vi "Pack for gRPC.vi"(8 "error in":errorcluster, 9 "configuration / results":enum16{"Configuration", "Results"}(ring), 10 "data value":variant, 11 "measurement customizations in":refnum<class "Measurement Plugin.lvclass">) -> (0 "error out":errorcluster, 2 "any":T1, 3 "measurement customizations out":refnum<class "Measurement Plugin.lvclass">)   [LabVIEW 2021, in "Waveform Mode_Channel Ganging.lvlib" / "Measurement Plugin.lvclass"]
uses:
  Measurement Plugin.lvclass
  <vilib>/gRPC/LabVIEW gRPC Library/Shared/Any.ctl
  C:/Program Files/National Instruments/LabVIEW 2021/vi.lib/Plug-In SDKs/Measurements/Measurement Plugin Service/Measurement Plugin Service.lvclass
  Measurement Configuration.ctl
  Measurement Results.ctl
  2eca732d-dbaa-43bf-a7dd-ede2da65bc1b.vi
  a6012965-5700-4384-8228-972e71b6560c.vi
  <vilib>/gRPC/LabVIEW gRPC Library/Server API/Translate Protobuf Error.vi
  <vilib>/AdvancedString/1D String Array to Delimited String.vi
  <vilib>/gRPC/LabVIEW gRPC Library/Server API/Server/Get Server DLL Path.vi
  Measurement Plugin.lvclass/Measurement Plugin.ctl
  Waveform Mode_Channel Ganging.lvlib
  <vilib>/Plug-In SDKs/Measurements/Measurement Plugin Service/Measurement Plugin Service.lvclass
  <vilib>/gRPC/LabVIEW gRPC Library/grpc-lvsupport-release.lvlib
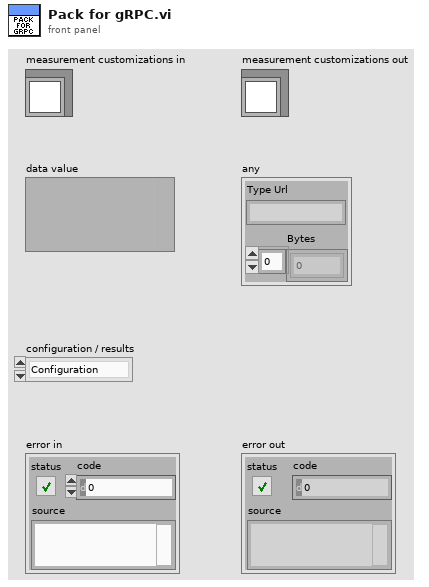
[diagram p1: front panel]
types:
  T1 = typedef "grpc-lvsupport-release.lvlib/Any.ctl" = cluster{"Type Url":string, "Bytes":u8[]}
  T2 = typedef "grpc-lvsupport-release.lvlib/grpcId.ctl" = u64
  T3 = typedef "Waveform Mode_Channel Ganging.lvlib/Measurement Configuration.ctl" = cluster{"Source voltage/current gain bandwidths":dbl[], "Source voltage/current compensation frequencies":dbl[], "Source voltage/current pole-zero ratios":dbl[], "Load voltage/current gain bandwidths":dbl[], "Load voltage/current compensation frequencies":dbl[], "Load voltage/current pole-zero ratios":dbl[], "Source enable/disable":bool, "Load enable/disable":bool, "Source master resource name":string, "Source slave resource names":string[], "Load master resource name":string, "Load slave resource names":string[], "Source voltage/current setpoints":dbl[], "Source source delays":dbl[], "Load voltage/current setpoints":dbl[], "Load source delays":dbl[], "Source system configuration":enum32{"Series", "Parallel", "Manual"}, "Source output function":i32, "Source voltage/current level range":dbl, "Source sense":i32, "Source limit symmetry":enum32{"Symmetric", "Asymmetric"}, "Source current/voltage limit range":dbl, "Source current/voltage limit low":dbl, "Source current/voltage limit high":dbl, "Source aperture time":dbl, "Source transient response":i32, "Load system configuration":enum32{"Series", "Parallel", "Manual"}, "Load output function":i32, "Load voltage/current level range":dbl, "Load sense":i32, "Load limit symmetry":enum32{"Symmetric", "Asymmetric"}, "Load current/voltage limit range":dbl, "Load current/voltage limit low":dbl, "Load current/voltage limit high":dbl, "Load aperture time":dbl, "Load transient response":i32, "Load source trigger":string, "Load measure trigger":string}
  T4 = typedef "Waveform Mode_Channel Ganging.lvlib/Measurement Results.ctl" = cluster{"Source dt":dbl[], "Source voltages":dbl[], "Source currents":dbl[], "Ganged source voltages":dbl[], "Ganged source currents":dbl[], "Load dt":dbl[], "Load voltages":dbl[], "Load currents":dbl[], "Ganged load voltages":dbl[], "Ganged load currents":dbl[]}
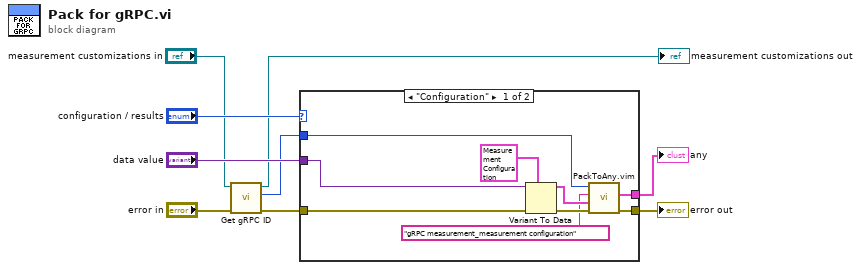
[diagram p0: block diagram]
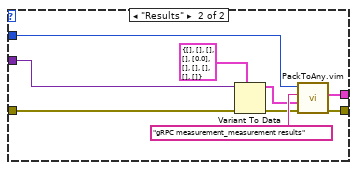
[diagram p2: hidden frame]
diagram:
  n1 = call <vilib>:"Get gRPC ID.vi"("error in"="error in", "measurement plugin service in"="measurement customizations in") -> ("error out"=w4:errorcluster, "gRPC ID"=w1:T2, "measurement plugin service out"=→"measurement customizations out":refnum<class "Measurement Plugin.lvclass">)  [unwired: 7 in]
  n2 = case shown="\"Configuration\"" "configuration / results" {
    tunnel: w4 -> [w18 w27]
    tunnel: "data value" -> [w17 w26]
    tunnel: w1 -> [w14 w22]
    tunnel: [w16 w24] -> w8
    tunnel: [w15 w23] -> w7
    frame "Configuration" {
      n3 = Variant To Data(error in=w18, type=T3 {"Source voltage/current gain bandwidths"=[], "Source voltage/current compensation frequencies"=[], "Source voltage/current pole-zero ratios"=[], "Load voltage/current gain bandwidths"=[], "Load voltage/current compensation frequencies"=[], "Load voltage/current pole-zero ratios"=[], "Source enable/disable"=TRUE, "Load enable/disable"=TRUE, "Source master resource name"="", "Source slave resource names"=[], "Load master resource name"="", "Load slave resource names"=[], "Source voltage/current setpoints"=[], "Source source delays"=[], "Load voltage/current setpoints"=[], "Load source delays"=[], "Source system configuration"=enum."Parallel", "Source output function"=1006, "Source voltage/current level range"=20.0, "Source sense"=1009, "Source limit symmetry"=enum."Asymmetric", "Source current/voltage limit range"=25.0, "Source current/voltage limit low"=-0.6, "Source current/voltage limit high"=25.0, "Source aperture time"=0.01666, "Source transient response"=1038, "Load system configuration"=enum."Parallel", "Load output function"=1007, "Load voltage/current level range"=80.0, "Load sense"=1009, "Load limit symmetry"=enum."Symmetric", "Load current/voltage limit range"=6.0, "Load current/voltage limit low"=0.0, "Load current/voltage limit high"=inf, "Load aperture time"=0.01666, "Load transient response"=1038, "Load source trigger"="", "Load measure trigger"=""} ("measurement configuration"), Variant=w17) -> (data=w13:T3, error out=w12:errorcluster)
      n4 = call "PackToAny.vim"("error in"=w12, "Data To Pack"=w13, "Message Type"="gRPC measurement_measurement configuration", "gRPCid in"=w14) -> ("error out"=w16:errorcluster, "Any"=w15:T1)  [unwired: 5 in, 1 out]
    }
    frame "Results" {
      n5 = Variant To Data(error in=w27, type=T4 {"Source dt"=[], "Source voltages"=[], "Source currents"=[], "Ganged source voltages"=[], "Ganged source currents"=[0.0], "Load dt"=[], "Load voltages"=[], "Load currents"=[], "Ganged load voltages"=[], "Ganged load currents"=[]} ("Measurement Results"), Variant=w26) -> (data=w20:T4, error out=w19:errorcluster)
      n6 = call "PackToAny.vim"("error in"=w19, "Data To Pack"=w20, "Message Type"="gRPC measurement_measurement results", "gRPCid in"=w22) -> ("error out"=w24:errorcluster, "Any"=w23:T1)  [unwired: 5 in, 1 out]
    }
  }
  "error out" <- w8
  "any" <- w7
